vi "W7X2DPut_Reduced.vi"(0 "SigLabel":string, 5 "SigJSONbuffer":string, 7 "values":T1(array[cluster]), 8 "dimensions":i64[](array[numeric])=[1399090569999999999, -1], 9 "sample rate":u16, 11 "sample period":dbl, 12 "pulse_length":dbl) -> (10 "file path written":string, 14 "Parlog error out":errorcluster)   [LabVIEW 2014]
uses:
  <vilib>/httpClient/POSTBuffer.vi
  <vilib>/httpClient/LabVIEWHTTPClient.lvlib
panel:
  out "JSON string":string
  out "body":string
  out "headers":string
  out "body Parlog":string
  out "headers parms":string
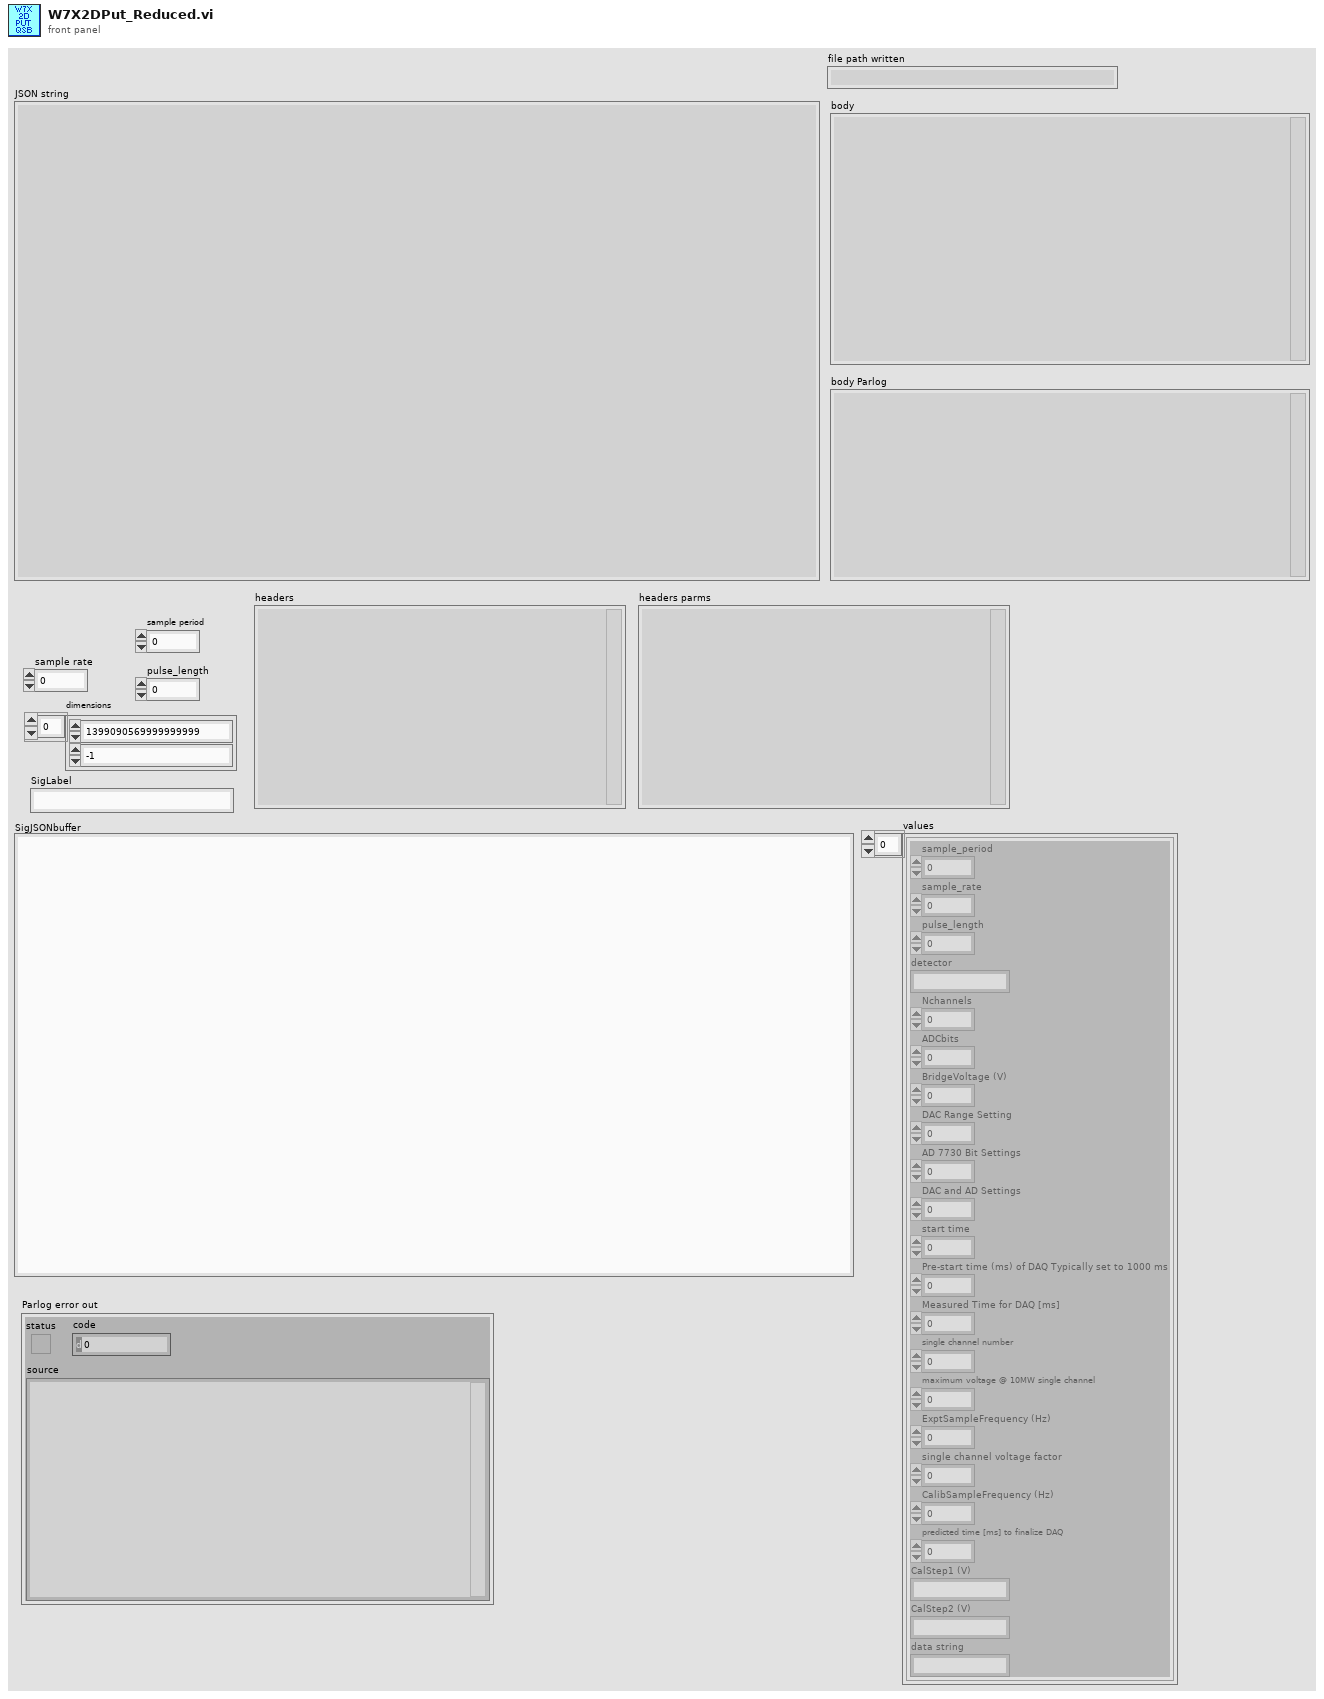
[diagram p1: front panel]
types:
  T1 = cluster{"sample_period":dbl, "sample_rate":dbl, "pulse_length":dbl, "detector":string, "Nchannels":i16, "ADCbits":i16, "BridgeVoltage (V)":sgl, "DAC Range Setting":u8, "AD 7730 Bit Settings":i32, "DAC and AD Settings":i32, "start time":i64, "Pre-start time (ms) of DAQ Typically set to 1000 ms":i32, "Measured Time for DAQ [ms] ":u32, "single channel number":i64, "maximum voltage @ 10MW single channel":dbl, "ExptSampleFrequency (Hz)":sgl, "single channel voltage factor":dbl, "CalibSampleFrequency (Hz)":sgl, "predicted time [ms] to finalize DAQ":dbl, "CalStep1 (V)":string, "CalStep2 (V)":string, "data string":string}[]
  T2 = cluster{"sample_period":dbl, "sample_rate":dbl, "pulse_length":dbl, "detector":string, "Nchannels":i16, "ADCbits":i16, "BridgeVoltage (V)":sgl, "DAC Range Setting":u8, "AD 7730 Bit Settings":i32, "DAC and AD Settings":i32, "start time":i64, "Pre-start time (ms) of DAQ Typically set to 1000 ms":i32, "Measured Time for DAQ [ms] ":u32, "single channel number":i64, "maximum voltage @ 10MW single channel":dbl, "ExptSampleFrequency (Hz)":sgl, "single channel voltage factor":dbl, "CalibSampleFrequency (Hz)":sgl, "predicted time [ms] to finalize DAQ":dbl, "CalStep1 (V)":string, "CalStep2 (V)":string, "data string":string}
  T3 = typedef "LabVIEWHTTPClient.lvlib/ClientHandle.ctl" = refnum<k1>
  T4 = cluster{"label":string, "values":cluster{"sample_period":dbl, "sample_rate":dbl, "pulse_length":dbl, "detector":string, "Nchannels":i16, "ADCbits":i16, "BridgeVoltage (V)":sgl, "DAC Range Setting":u8, "AD 7730 Bit Settings":i32, "DAC and AD Settings":i32, "start time":i64, "Pre-start time (ms) of DAQ Typically set to 1000 ms":i32, "Measured Time for DAQ [ms] ":u32, "single channel number":i64, "maximum voltage @ 10MW single channel":dbl, "ExptSampleFrequency (Hz)":sgl, "single channel voltage factor":dbl, "CalibSampleFrequency (Hz)":sgl, "predicted time [ms] to finalize DAQ":dbl, "CalStep1 (V)":string, "CalStep2 (V)":string, "data string":string}[], "dimensions":i64[]}
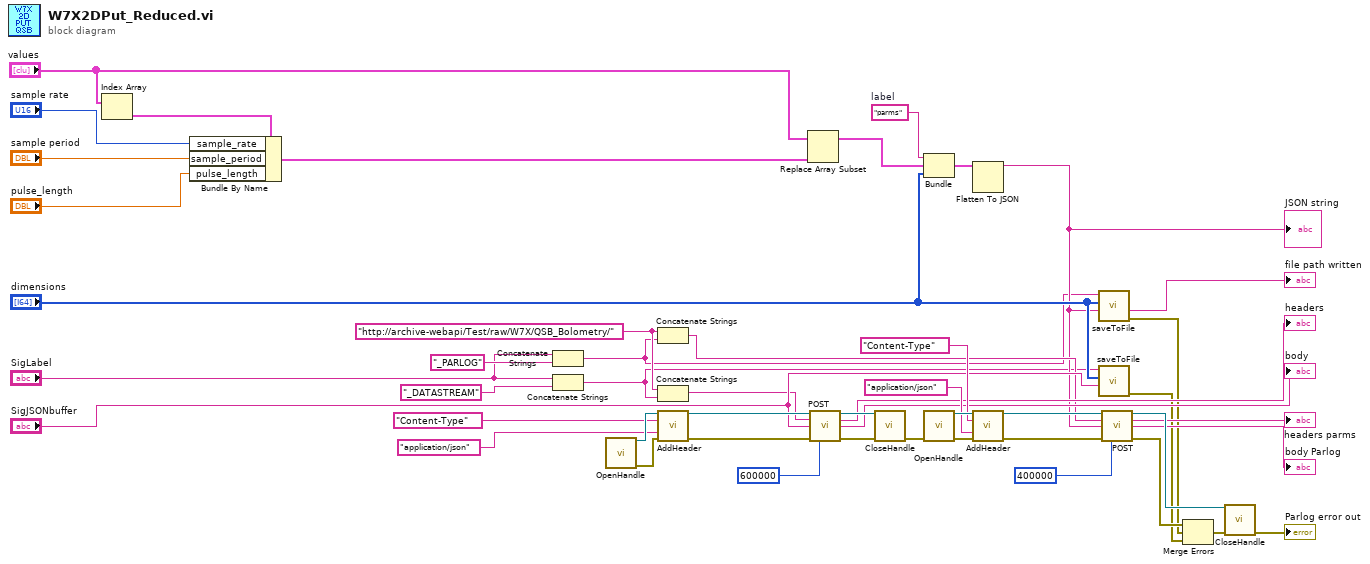
[diagram p0: block diagram]
diagram:
  w23 = "parms"  # label
  w13 = "http://archive-webapi/Test/raw/W7X/QSB_Bolometry/" ("url")
  n1 = Index Array(array="values") -> (element=w18:T2)  [unwired: 1 in]
  n2 = Bundle By Name(cluster=w18, "sample_rate"="sample rate", "sample_period"="sample period", "pulse_length"="pulse_length") -> (w1:T2)
  n3 = Concatenate Strings("SigLabel", "_PARLOG" ("replace string (\"\")")) -> (w6:string)
  n4 = Concatenate Strings("SigLabel", "_DATASTREAM" ("string")) -> (w5:string)
  n5 = call <vilib>:"OpenHandle.vi"() -> ("client handle out"=w33:T3, "error out"=w32:errorcluster)  [unwired: 14 in]
  n6 = Concatenate Strings(w13, w6) -> (w14:string)
  n7 = Concatenate Strings(w13, w5) -> (w3:string)
  n8 = call <vilib>:"AddHeader.vi"("client handle"=w33, "header"="Content-Type", "value"="application/json", "error in (no error)"=w32) -> ("client handle out"=w31:T3, "error out"=w30:errorcluster)  [unwired: 10 in]
  n9 = Replace Array Subset(array="values", new element=w1) -> (w17:T1)  [unwired: 1 in]
  n10 = call-poly <vilib>:"POST.vi"("client handle"=w31, "url"=w3, "buffer"="SigJSONbuffer", "error in (no error)"=w30, "timeout (10000)"=600000) -> ("client handle out"=w36:T3, "headers"=→"headers":string, "body"=→"body":string, "error out"=w35:errorcluster)  [unwired: 7 in]
  n11 = call <vilib>:"CloseHandle.vi"("client handle"=w36, "error in (no error)"=w35) -> ("error out"=w7:errorcluster)  [unwired: 13 in]
  n12 = Bundle("label"=w23, "values"=w17, "dimensions"="dimensions") -> (w22:T4)  [unwired: 1 in]
  n13 = call <vilib>:"OpenHandle.vi"("error in (no error)"=w7) -> ("client handle out"=w45:T3, "error out"=w44:errorcluster)  [unwired: 13 in]
  n14 = Flatten To JSON(anything=w22) -> (JSON string=w11:string)  [unwired: 2 in, 1 out]
  "JSON string" <- w11
  n15 = call <vilib>:"AddHeader.vi"("client handle"=w45, "header"="Content-Type", "value"="application/json", "error in (no error)"=w44) -> ("client handle out"=w43:T3, "error out"=w42:errorcluster)  [unwired: 10 in]
  n16 = call "saveToFile.vi"("SigJSONbuffer"=w11, "dimensions"="dimensions", "String"=w6) -> ("error out"=w9:errorcluster, "resulting string"=→"file path written":string)  [unwired: 7 in]
  n17 = call "saveToFile.vi"("SigJSONbuffer"="SigJSONbuffer", "dimensions"="dimensions", "String"=w5) -> ("error out"=w8:errorcluster)  [unwired: 7 in, 1 out]
  n18 = call-poly <vilib>:"POST.vi"("client handle"=w43, "url"=w14, "buffer"=w11, "error in (no error)"=w42, "timeout (10000)"=400000) -> ("client handle out"=w48:T3, "headers"=→"headers parms":string, "body"=→"body Parlog":string, "error out"=w47:errorcluster)  [unwired: 7 in]
  n19 = Merge Errors(w47, w9, w8) -> (w10:errorcluster)
  n20 = call <vilib>:"CloseHandle.vi"("client handle"=w48, "error in (no error)"=w10) -> ("error out"=→"Parlog error out":errorcluster)  [unwired: 13 in]
